vi "Finish Part.vi"(8 "error in (no error)":errorcluster, 11 "Multipart Parser in":refnum<class "Multipart Parser.lvclass">) -> (0 "error out":errorcluster, 3 "Multipart Parser out":refnum<class "Multipart Parser.lvclass">)   [LabVIEW 2020, in "HTTP Utils.lvlib" / "Multipart Parser.lvclass"]
uses:
  Multipart Parser.lvclass
  Multipart Parser.lvclass/Multipart Parser.ctl
  Request/Request.lvclass
  FormField/FormField.lvclass
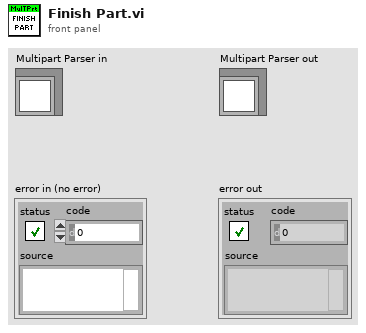
[diagram p1: front panel]
types:
  T1 = typedef "HTTP Utils.lvlib/Request.lvclass/Content-Disposition.ctl" = cluster{"Type":string, "Name":string, "Filename":string}
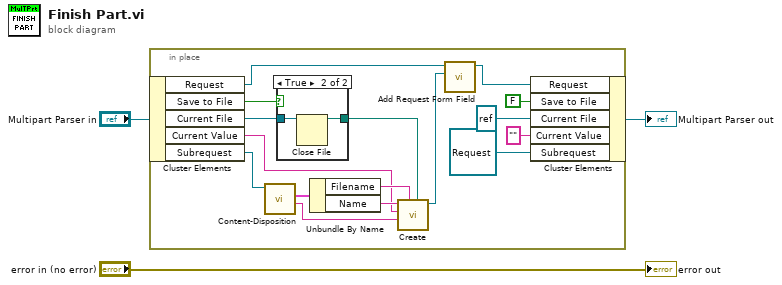
[diagram p0: block diagram]
diagram:
  n1 = in-place {
    n2 = in-place-cluster #1("Multipart Parser in") -> ("Request"=w6:refnum<class "Request.lvclass">, "Save to File"=w9:bool, "Current File"=w10:refnum<file>, "Current Value"=w11:string, "Subrequest"=w17:refnum<class "Request.lvclass">)
    n3 = call "Content-Disposition.vi"("Request in"=w17) -> ("Content-Type"=w12:string, "Content-Disposition"=w16:T1)  [unwired: 6 in, 3 out]
    n4 = case shown="True" w9 {
      tunnel: [_ w21] -> w13
      tunnel: w10 -> [_ w20]
      frame False {
      }
      frame True {
        n5 = Close File(refnum=w20) -> (path=w21:path)  [unwired: 1 in, 1 out]
      }
    }
    n6 = Unbundle By Name(w16) -> ("Filename"=w14:string, "Name"=w15:string)
    n7 = call "Create.vi"("File Path"=w13, "Original Name"=w14, "MIME Type"=w12, "Value"=w11, "Name"=w15) -> ("FormField"=w5:refnum<class "FormField.lvclass">)  [unwired: 6 in]
    n8 = call "Add Request Form Field.vi"("FormField"=w5, "Request in"=w6) -> ("Request out"=w4:refnum<class "Request.lvclass">)  [unwired: 8 in, 1 out]
    n9 = in-place-cluster #1("Request"=w4, "Save to File"=FALSE, "Current File"=refnum<file> refnum, "Current Value"="", "Subrequest"=refnum<class "Request.lvclass"> refnum) -> (→"Multipart Parser out":refnum<class "Multipart Parser.lvclass">)
  }
  "error out" <- "error in (no error)"
